vi "AG34980A ESE.vi"(0 "VISA resource name":refnum<visa-resource-name>, 11 "error in (no error)":errorcluster) -> (4 "VISA resource name out":refnum<visa-resource-name>, 6 "x != 0?":bool, 10 "ESE Message":string, 15 "error out":errorcluster)   [LabVIEW 2009]
doc: "This VI reads an error from the instrument. It expects to see errors in SCPI format (#,\"error message\"). If an error query is not supported, it returns a warning."
panel:
  out "return count":u32
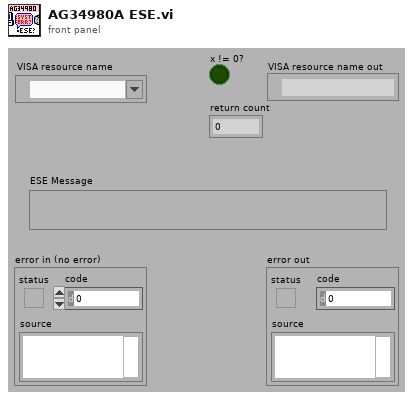
[diagram p1: front panel]
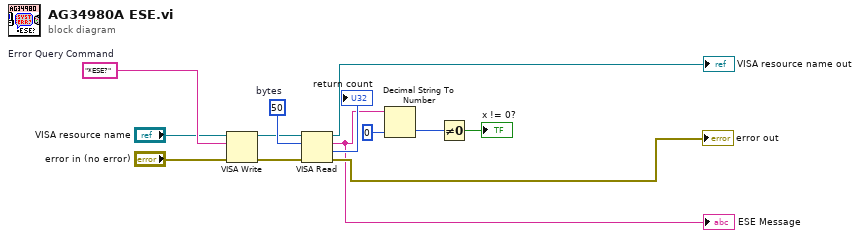
[diagram p0: block diagram]
diagram:
  w11 = u32 50  # bytes
  w7 = "*ESE?"  # Error Query Command
  n1 = VISA Write(VISA resource name="VISA resource name", write buffer=w7, error in (no error)="error in (no error)") -> (VISA resource name out=w10:refnum<visa-resource-name>, error out=w12:errorcluster)  [unwired: 1 out]
  n2 = VISA Read(VISA resource name=w10, byte count=w11, error in (no error)=w12) -> (VISA resource name out=→"VISA resource name out":refnum<visa-resource-name>, read buffer=w2:string, return count=→"return count":u32, error out=→"error out":errorcluster)
  "ESE Message" <- w2
  n3 = Decimal String To Number(string=w2, default (0L)=0) -> (number=w9:i32)  [unwired: 1 in, 1 out]
  n4 = Not Equal To 0?(x=w9) -> (x != 0?=→"x != 0?":bool)
